vi "UDP - Data Sensor (SubVI).vi"(8 "error in":errorcluster, 11 "String":string="\u0002”<wy02 25\u0000\u0000\u0000mm\u0000\u0000\u0000\u0000\u0003\u0000\u0000\u0000\u0000\u0000ÈA\u0000\u0000\u0000\u0000\u000f\u0000\u0000\u0000\u0007\u0000\u0000\u0000Disp.\u0000\u0000\u0000\u0000\u0000mm\u0000\u0000\u0000\u0000\u0003p.1\u0000\u0000\u0000\u0000mm\u0000\u0000\u0001\u0000\u0000\u0000\u0002\u0000\u0000\u0000Ch3\u0000\u0000\u0000\u0000\u0000\u0000\u0000Unit\u0000\u0000\u0002\u0000\u0000\u0000\u0000\u0000\u0000\u0000\u0000\u0001\u0002\u0002\u0001\u0000\u0000\u0000\u0002\u0000\u0000\u0000Ch4\u0000\u0000\u0000\u0000\u0000\u0000\u0000Unit\u0000\u0000\u0002\u0000\u0000\u0000\u0000\u0000\u0000\u0000\u0000\u0000\u0000\u0000\u0001\u0000\u0000\u0000\u0002\u0000\u0000\u0000h") -> (0 "error out":errorcluster, 3 "Sensor Out":T1, 4 "Success":bool)   [LabVIEW 2019]
panel:
  in  "String 2":string="\u0002”<wy02 25\u0000\u0000\u0000mm\u0000\u0000\u0000\u0000\u0003\u0000\u0000\u0000\u0000\u0000ÈA\u0000\u0000\u0000\u0000\u000f\u0000\u0000\u0000\u0007\u0000\u0000\u0000Disp.\u0000\u0000\u0000\u0000\u0000mm\u0000\u0000\u0000\u0000\u0003p.1\u0000\u0000\u0000\u0000mm\u0000\u0000\u0001\u0000\u0000\u0000\u0002\u0000\u0000\u0000Ch3\u0000\u0000\u0000\u0000\u0000\u0000\u0000Unit\u0000\u0000\u0002\u0000\u0000\u0000\u0000\u0000\u0000\u0000\u0000\u0001\u0002\u0002\u0001\u0000\u0000\u0000\u0002\u0000\u0000\u0000Ch4\u0000\u0000\u0000\u0000\u0000\u0000\u0000Unit\u0000\u0000\u0002\u0000\u0000\u0000\u0000\u0000\u0000\u0000\u0000\u0000\u0000\u0000\u0001\u0000\u0000\u0000\u0002\u0000\u0000\u0000h"
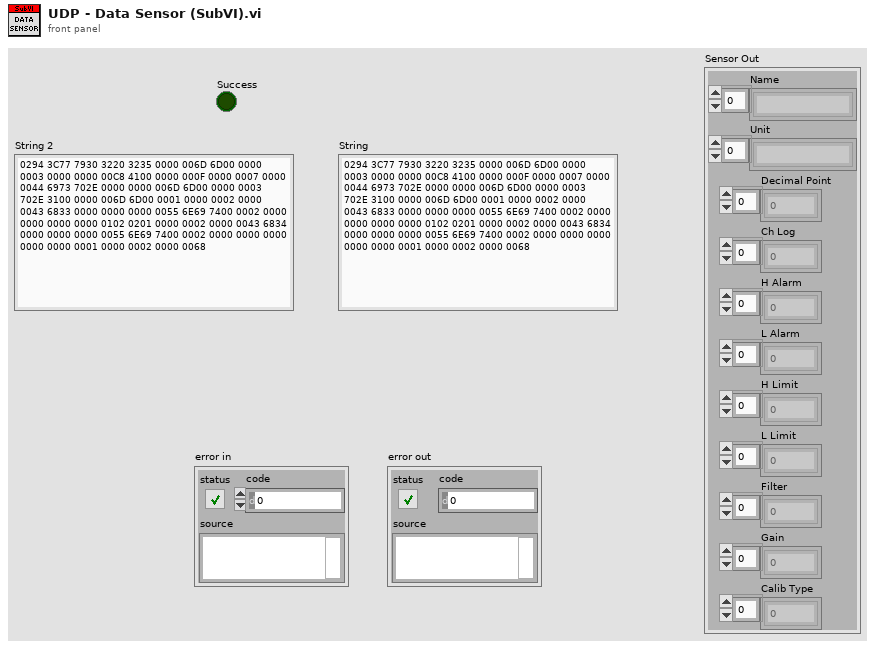
[diagram p1: front panel]
types:
  T1 = cluster{"Name":string[], "Unit":string[], "Decimal Point":u8[], "Ch Log":u8[], "H Alarm":u8[], "L Alarm":u8[], "H Limit":sgl[], "L Limit":sgl[], "Filter":u8[], "Gain":u8[], "Calib Type":u32[]}
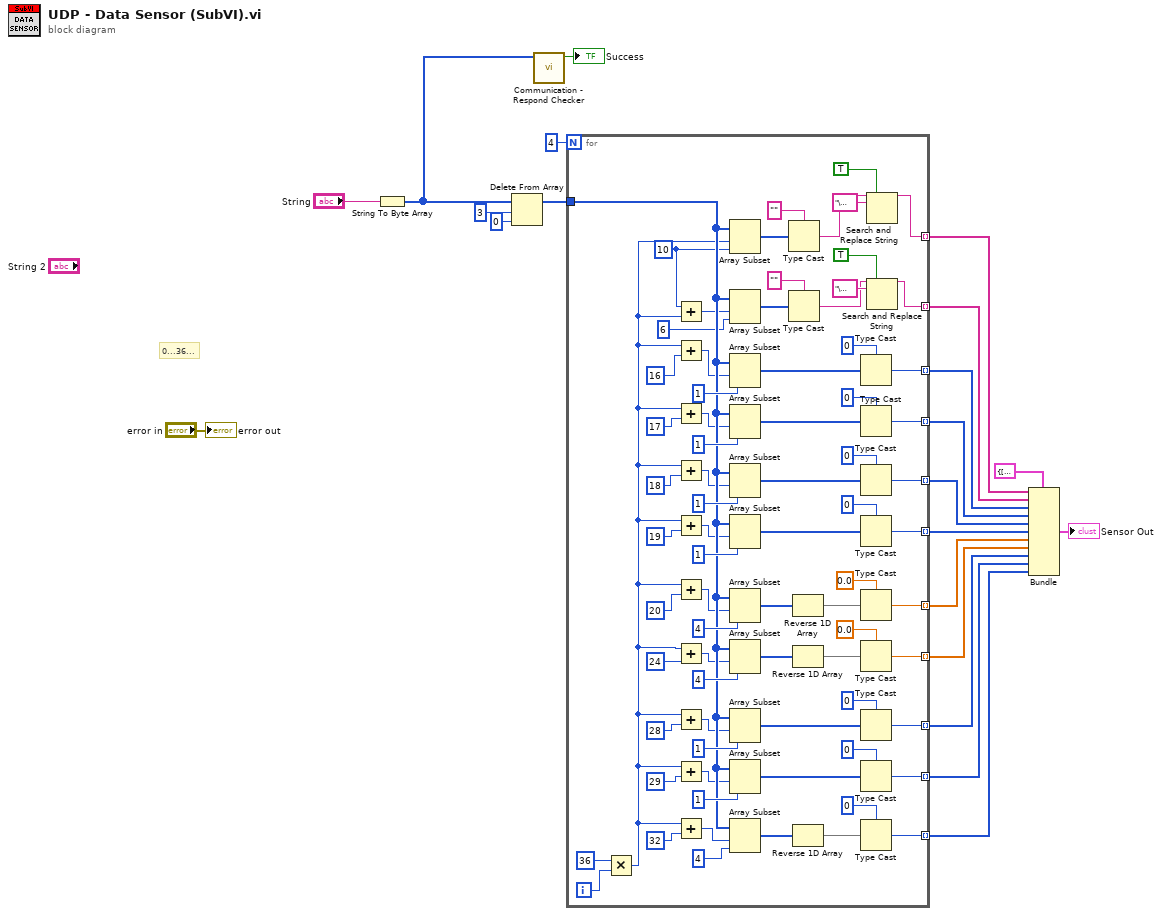
[diagram p0: block diagram]
diagram:
  # "0...36..."
  n1 = String To Byte Array(string="String") -> (unsigned byte array=w16:u8[])
  n2 = Delete From Array(array=w16, length=3, index=0) -> (array with subset deleted=w19:u8[])  [unwired: 1 out]
  n3 = call "Communication - Respond Checker.vi"("Read Data"=w16) -> ("Success"=→"Success":bool)  [unwired: 10 in]
  n4 = for {
    N: 4 -> [_]
    tunnel: w19 -> [w63]
    tunnel: [w38] -> w3 mode=indexing
    tunnel: [w37] -> w4 mode=indexing
    tunnel: [w36] -> w5 mode=indexing
    tunnel: [w35] -> w6 mode=indexing
    tunnel: [w34] -> w7 mode=indexing
    tunnel: [w33] -> w8 mode=indexing
    tunnel: [w32] -> w9 mode=indexing
    tunnel: [w31] -> w10 mode=indexing
    tunnel: [w30] -> w11 mode=indexing
    tunnel: [w22] -> w12 mode=indexing
    tunnel: [w28] -> w13 mode=indexing
    i -> [w62]
    w60 = 10 ("length")
    n5 = Multiply(x=36, y=w62) -> (x*y=w40:i32)
    n6 = Add(x=w60, y=w40) -> (x+y=w59:i32)
    n7 = Add(x=w40, y=16 ("index")) -> (x+y=w56:i32)
    n8 = Add(x=w40, y=17 ("index")) -> (x+y=w54:i32)
    n9 = Add(x=w40, y=18 ("index")) -> (x+y=w52:i32)
    n10 = Add(x=w40, y=19 ("index")) -> (x+y=w50:i32)
    n11 = Add(x=w40, y=20 ("index")) -> (x+y=w48:i32)
    n12 = Add(x=w40, y=24 ("index")) -> (x+y=w46:i32)
    n13 = Add(x=w40, y=28 ("index")) -> (x+y=w44:i32)
    n14 = Add(x=w40, y=29 ("index")) -> (x+y=w42:i32)
    n15 = Add(x=w40, y=32 ("index")) -> (x+y=w39:i32)
    n16 = Array Subset(array=w63, index=w40, length=w60) -> (w92:u8[])
    n17 = Array Subset(array=w63, index=w59, length=6) -> (w91:u8[])
    n18 = Array Subset(array=w63, index=w56, length=1) -> (w90:u8[])
    n19 = Array Subset(array=w63, index=w54, length=1) -> (w89:u8[])
    n20 = Array Subset(array=w63, index=w52, length=1) -> (w87:u8[])
    n21 = Array Subset(array=w63, index=w50, length=1) -> (w88:u8[])
    n22 = Array Subset(array=w63, index=w48, length=4) -> (w78:u8[])
    n23 = Array Subset(array=w63, index=w46, length=4) -> (w77:u8[])
    n24 = Array Subset(array=w63, index=w44, length=1) -> (w69:u8[])
    n25 = Array Subset(array=w63, index=w42, length=1) -> (w68:u8[])
    n26 = Array Subset(array=w63, index=w39, length=4) -> (w67:u8[])
    n27 = Type Cast(type="", x=w92) -> (*(type *) &x=w29:string)
    n28 = Type Cast(type="", x=w91) -> (*(type *) &x=w23:string)
    n29 = Reverse 1D Array(array=w78) -> (reversed array=w76:u8[])
    n30 = Reverse 1D Array(array=w77) -> (reversed array=w75:u8[])
    n31 = Reverse 1D Array(array=w67) -> (reversed array=w66:u8[])
    n32 = Type Cast(type=u8 0, x=w90) -> (*(type *) &x=w30:u8)
    n33 = Type Cast(type=u8 0, x=w89) -> (*(type *) &x=w31:u8)
    n34 = Type Cast(type=u8 0, x=w87) -> (*(type *) &x=w32:u8)
    n35 = Type Cast(type=u8 0, x=w88) -> (*(type *) &x=w33:u8)
    n36 = Type Cast(type=sgl 0.0, x=w76) -> (*(type *) &x=w34:sgl)
    n37 = Type Cast(type=sgl 0.0, x=w75) -> (*(type *) &x=w35:sgl)
    n38 = Type Cast(type=u8 0, x=w69) -> (*(type *) &x=w36:u8)
    n39 = Type Cast(type=u8 0, x=w68) -> (*(type *) &x=w37:u8)
    n40 = Type Cast(type=u32 0, x=w66) -> (*(type *) &x=w38:u32)
    n41 = Search and Replace String(replace all?=TRUE ("replace all? (F)"), input string=w29, search string="\u0000") -> (result string=w28:string)  [unwired: 5 in, 3 out]
    n42 = Search and Replace String(replace all?=TRUE ("replace all? (F)"), input string=w23, search string="\u0000") -> (result string=w22:string)  [unwired: 5 in, 3 out]
  }
  n43 = Bundle(cluster=T1 {"Name"=[], "Unit"=[], "Decimal Point"=[], "Ch Log"=[], "H Alarm"=[], "L Alarm"=[], "H Limit"=[], "L Limit"=[], "Filter"=[], "Gain"=[], "Calib Type"=[]} ("output cluster"), "Name"=w13, "Unit"=w12, "Decimal Point"=w11, "Ch Log"=w10, "H Alarm"=w9, "L Alarm"=w8, "H Limit"=w7, "L Limit"=w6, "Filter"=w5, "Gain"=w4, "Calib Type"=w3) -> (→"Sensor Out":T1)
  "error out" <- "error in"
